vi "HBDecode.vi"(0 "handle":u64, 5 "pSrcData":u8[](array[numeric]), 7 "pDstBuf In":u8[](array[numeric]), 9 "SrcDataLen":u32, 11 "error in (no error)":errorcluster caption="错误输入（无错误）", 12 "DstBufferSize":u32) -> (4 "handle out":u64, 6 "function return":i32 format="%x", 8 "pDstBuf Out":u8[](array[numeric]), 10 "pHBDecode Out":T1, 15 "error out":errorcluster caption="错误输出")   [LabVIEW 2013, in "MvCameraControl.lvlib"]
doc: "MV_CAMPAT_API int __stdcall MV_CP_ConvertPixelType();"
uses:
  MvCameraControl.lvlib
  MvCameraPatch.dll
panel:
  in  "pHBDecode In":T1
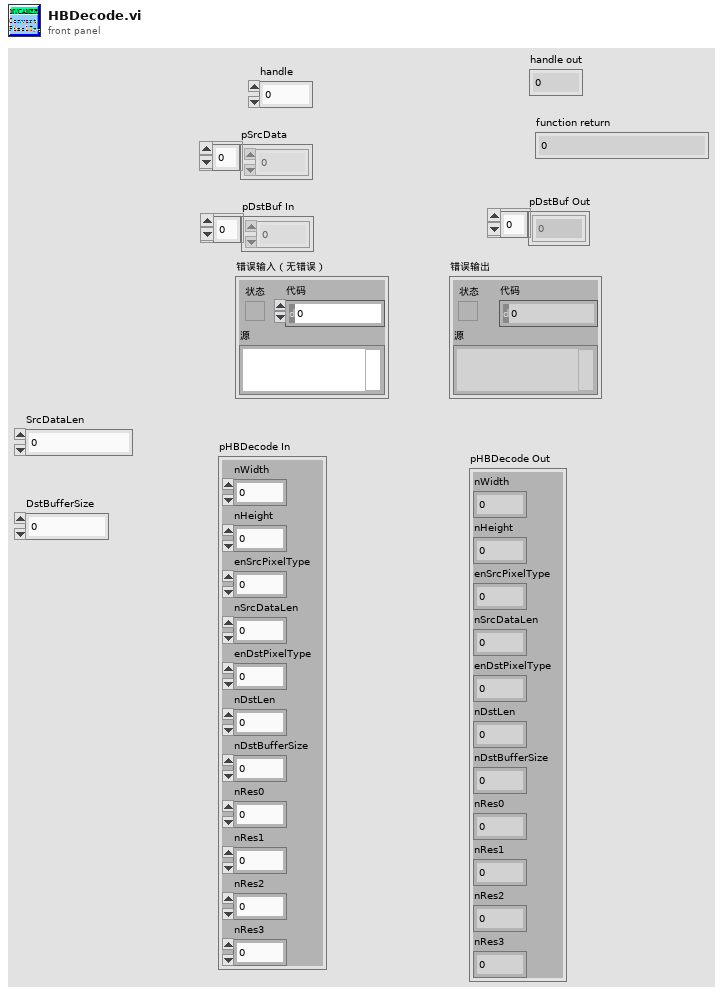
[diagram p1: front panel]
types:
  T1 = cluster{"nWidth":u32, "nHeight":u32, "enSrcPixelType":u32, "nSrcDataLen":u32, "enDstPixelType":u32, "nDstLen":u32, "nDstBufferSize":u32, "nRes0":u32, "nRes1":u32, "nRes2":u32, "nRes3":u32}
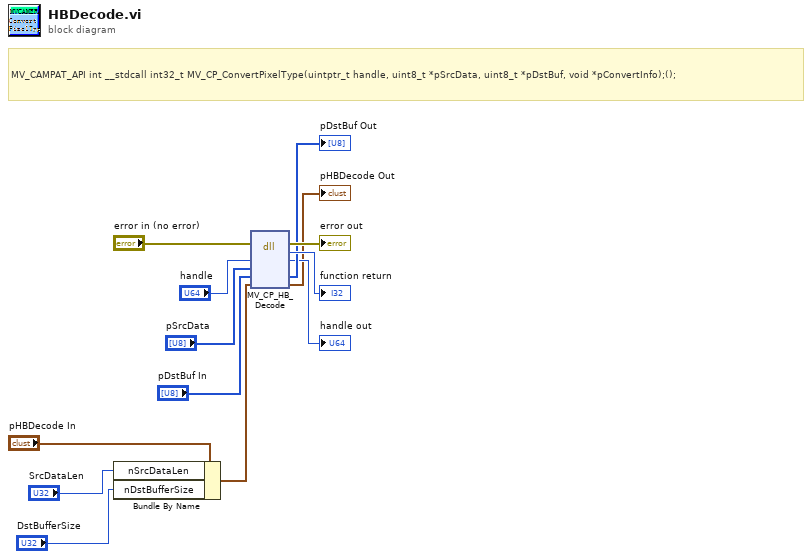
[diagram p0: block diagram]
diagram:
  # "MV_CAMPAT_API int __stdcall int32_t MV_CP_ConvertPixelType(uintptr_t handle, uint8_t *pSrcData, uint8_t *pDstBuf, void *pConvertInfo);();"
  n1 = Bundle By Name(cluster="pHBDecode In", "nSrcDataLen"="SrcDataLen", "nDstBufferSize"="DstBufferSize") -> (w4:T1)
  n2 = dll-call lib="MvCameraPatch.dll" fn="MV_CP_HB_Decode"(error in="error in (no error)", "handle"="handle", "pSrcData"="pSrcData", "pDstBuf"="pDstBuf In", "pHBDecodeInfo"=w4) -> (error out=→"error out":errorcluster, "返回类型"=→"function return":i32, "handle"=→"handle out":u64, "pDstBuf"=→"pDstBuf Out":u8[], "pHBDecodeInfo"=→"pHBDecode Out":T1)  [unwired: 3 in, 1 out]
